vi "newImageStringEvent.vi"(8 "error in (no error)":errorcluster, 9 "firstImage?":bool, 10 "ImageString":string, 11 "ImageStreamViewer in":refnum<class "ImageStreamViewer.lvclass">) -> (0 "error out":errorcluster, 3 "ImageStreamViewer out":refnum<class "ImageStreamViewer.lvclass">)   [LabVIEW 2011, in "Views.lvlib" / "Camera.lvlib" / "ImageStreamViewer.lvclass"]
uses:
  ImageStreamViewer.lvclass
  ImageStreamViewer.lvclass/ImageStreamViewer.ctl
panel:
  # "a new image string has arrived. \nWe need to unflatten it, and extract \nthe image information. then display it"
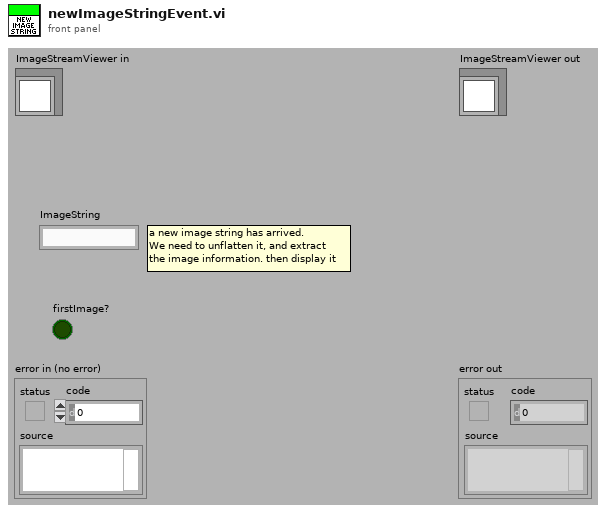
[diagram p1: front panel]
types:
  T1 = typedef "IMAQ Image.ctl" = refnum<image>
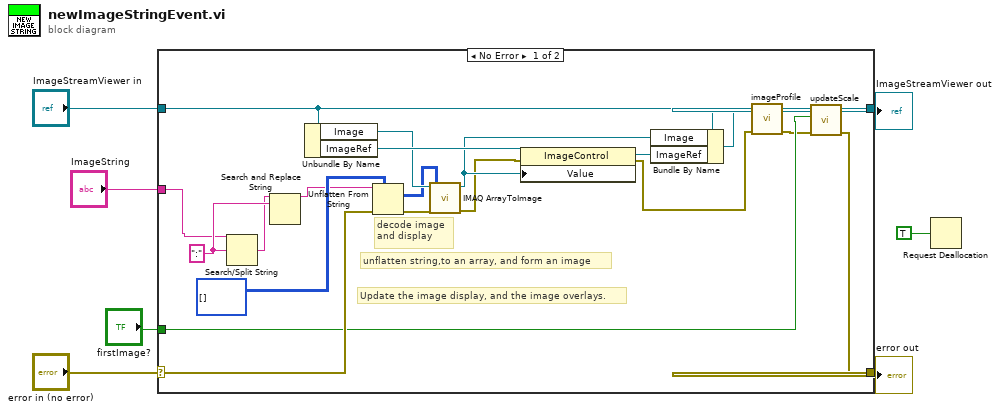
[diagram p0: block diagram]
diagram:
  n1 = case shown="No Error" "error in (no error)" {
    selector: "error in (no error)" -> [w28 w30]
    tunnel: [w8 w30] -> w6
    tunnel: [w12 w29] -> w4
    tunnel: "ImageStreamViewer in" -> [w25 w29]
    tunnel: "ImageString" -> [w21 _]
    tunnel: "firstImage?" -> [w10 _]
    frame No Error {
      w23 = ":"
      # "Update the image display, and the image overlays."
      # "unflatten string,to an array, and form an image"
      # "decode image\nand display"
      n2 = Search/Split String(string=w21, search string/char (-)=w23) -> (match + rest of string=w22:string)  [unwired: 1 in, 2 out]
      n3 = Search and Replace String(input string=w22, search string=w23) -> (result string=w20:string)  [unwired: 6 in, 3 out]
      n4 = Unbundle By Name(w25) -> ("Image"=w14:T1, "ImageRef"=w27:refnum<vi>)
      n5 = Unflatten From String(type=u16[][] [] ("Image data"), binary string=w20, error in (no error)=w28) -> (value=w13:u16[][], error out=w17:errorcluster)  [unwired: 2 in, 1 out]
      n6 = call "IMAQ ArrayToImage"("Image Pixels (U16)"=w13, "error in (no error)"=w17, "Image"=w14) -> ("error out"=w15:errorcluster, "Image Out"=w16:T1)  [unwired: 7 in]
      n7 = property class="ImageControl"(reference=w27, error in=w15, "Value"=w16) -> (reference out=w26:refnum<vi>, error out=w18:errorcluster)
      n8 = Bundle By Name(cluster=w25, "Image"=w16, "ImageRef"=w26) -> (w19:refnum<class "ImageStreamViewer.lvclass">)
      n9 = call "imageProfile.vi"("error in (no error)"=w18, "ImageStreamViewer in"=w19) -> ("error out"=w9:errorcluster, "ImageStreamViewer out"=w11:refnum<class "ImageStreamViewer.lvclass">)  [unwired: 8 in]
      n10 = call "updateScale.vi"("error in (no error)"=w9, "firstImage?"=w10, "ImageStreamViewer in"=w11) -> ("error out"=w8:errorcluster, "ImageStreamViewer out"=w12:refnum<class "ImageStreamViewer.lvclass">)  [unwired: 7 in]
    }
    frame Error {
    }
  }
  "error out" <- w6
  "ImageStreamViewer out" <- w4
  n11 = Request Deallocation(TRUE ("flag")) -> ()
